vi "ValueAsDateTime.vi"(8 "error in (no error)":errorcluster, 11 "Parameter":string="  <value><int>123</int></value>\n    ") -> (0 "error out":errorcluster, 3 "value":string)   [LabVIEW 2009]
doc: "Unpack ISO8601 Dat-Time string from XML-RPC format"
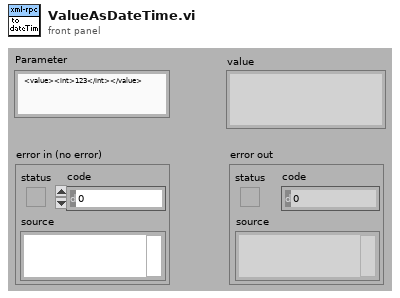
[diagram p1: front panel]
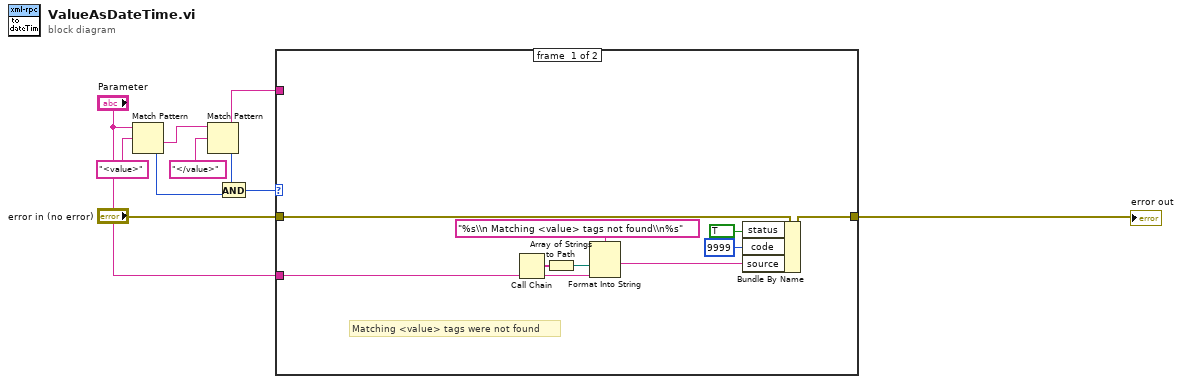
[diagram p0: block diagram]
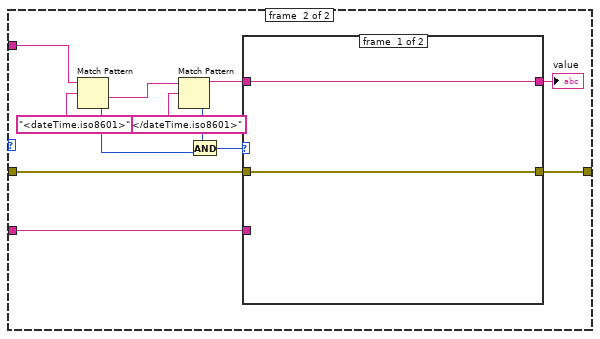
[diagram p2: hidden frame]
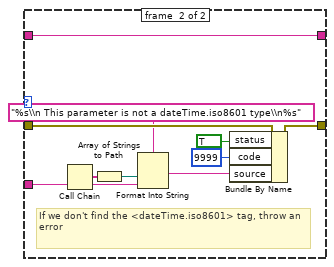
[diagram p3: hidden frame]
diagram:
  n1 = Match Pattern(string="Parameter", regular expression="<value>") -> (after substring=w9:string, offset past match=w2:i32)  [unwired: 1 in, 2 out]
  n2 = Match Pattern(string=w9, regular expression="</value>") -> (before substring=w7:string, offset past match=w3:i32)  [unwired: 1 in, 2 out]
  n3 = And(x=w3, y=w2) -> (x .and. y?=w1:i32)
  n4 = case shown="Default" w1 {
    tunnel: w7 -> [_ w28]
    tunnel: "error in (no error)" -> [w13 w26]
    tunnel: [w12 w20] -> w5
    tunnel: "Parameter" -> [w16 w25]
    frame #0 {
      # "Matching <value> tags were not found"
      n5 = Call Chain() -> (call chain=w19:string[])
      n6 = Array of Strings to Path(0:w19) -> (2:w18:path)  [unwired: 1 in]
      n7 = Format Into String(format string="%s\\n Matching <value> tags not found\\n%s", w18, w16) -> (resulting string=w11:string)  [unwired: 2 in, 1 out]
      n8 = Bundle By Name(cluster=w13, "status"=TRUE, "code"=9999, "source"=w11) -> (w12:errorcluster)
    }
    frame #1 {
      n9 = Match Pattern(string=w28, regular expression="<dateTime.iso8601>") -> (after substring=w30:string, offset past match=w23:i32)  [unwired: 1 in, 2 out]
      n10 = Match Pattern(string=w30, regular expression="</dateTime.iso8601>") -> (before substring=w27:string, offset past match=w24:i32)  [unwired: 1 in, 2 out]
      n11 = And(x=w24, y=w23) -> (x .and. y?=w22:i32)
      n12 = case shown="-1" w22 {
        tunnel: w27 -> [w33 w40]
        tunnel: [w33 w40] -> w21
        tunnel: w26 -> [w32 w43]
        tunnel: [w32 w42] -> w20
        tunnel: w25 -> [_ w41]
        frame #0 {
        }
        frame #1 {
          # "If we don't find the <dateTime.iso8601> tag, throw an error"
          n13 = Call Chain() -> (call chain=w39:string[])
          n14 = Array of Strings to Path(0:w39) -> (2:w36:path)  [unwired: 1 in]
          n15 = Format Into String(format string="%s\\n This parameter is not a dateTime.iso8601 type\\n%s", w36, w41) -> (resulting string=w35:string)  [unwired: 2 in, 1 out]
          n16 = Bundle By Name(cluster=w43, "status"=TRUE, "code"=9999, "source"=w35) -> (w42:errorcluster)
        }
      }
      "value" <- w21
    }
  }
  "error out" <- w5
